vi "Galvo-Control-V2.vi"() -> ()   [LabVIEW 2024]
uses:
  <vilib>/DAQmx/write.llb/DAQmx Write (Analog 1D DBL NChan 1Samp).vi
  <vilib>/DAQmx/create/channels.llb/DAQmx Create Channel (AO-Voltage-Basic).vi
  <vilib>/DAQmx/miscellaneous.llb/DAQmx Fill In Error Info.vi
panel:
  in  "Y desired voltage step(V/100)":dbl=1.0 format="%#_13g"
  in  "X desired voltage step(V/100)":dbl=1.0 format="%#_13g"
  out "Virtual Y position":dbl(graph)
  out "virtual X position":dbl(graph)
  out "Y indic":dbl
  out "X indic.":dbl
  in  "Y origin":dbl
  in  "X origin":dbl
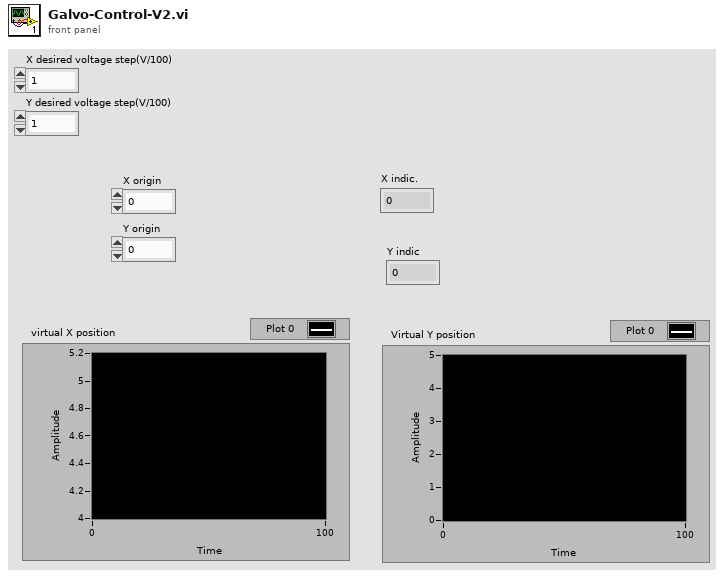
[diagram p1: front panel]
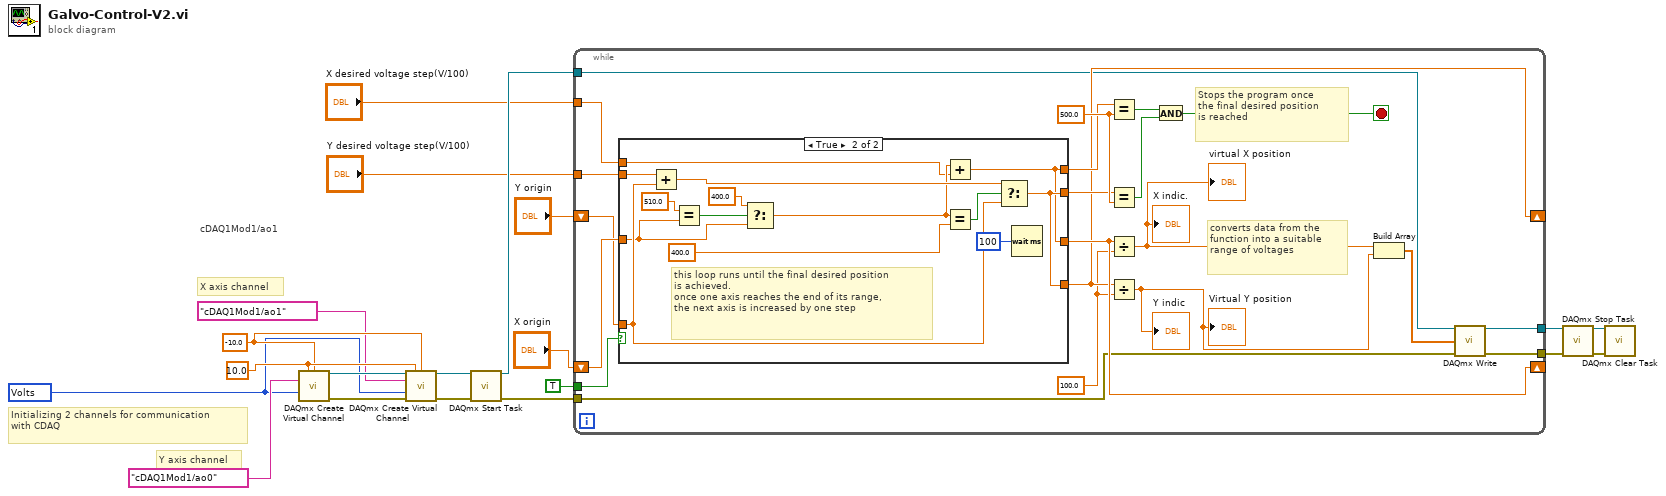
[diagram p0: block diagram]
diagram:
  w8 = 10348 items=["Volts"=10348, "From Custom Scale"=10065] ("units")
  w12 = 10.0 ("maximum value")
  w11 = -10.0 ("minimum value")
  # "Initializing 2 channels for communication\nwith CDAQ"
  # "cDAQ1Mod1/ao1"
  # "X axis channel"
  # "Y axis channel"
  n1 = call-poly <vilib>:"DAQmx Create Virtual Channel.vi"("maximum value"=w12, "minimum value"=w11, "physical channels"=tag "cDAQ1Mod1/ao0", "units"=w8) -> ("task out"=w18:refnum<k21>, "error out"=w17:errorcluster)  [unwired: 10 in]
  n2 = call-poly <vilib>:"DAQmx Create Virtual Channel.vi"("task in"=w18, "maximum value"=w12, "minimum value"=w11, "physical channels"=tag "cDAQ1Mod1/ao1", "units"=w8, "error in"=w17) -> ("task out"=w7:refnum<k21>, "error out"=w6:errorcluster)  [unwired: 8 in]
  n3 = call <vilib>:"DAQmx Start Task.vi"("task/channels in"=w7, "error in"=w6) -> ("task out"=w5:refnum<k21>, "error out"=w4:errorcluster)  [unwired: 12 in]
  n4 = while {
    shift-right: [w32] -> _
    shift-left: "X origin" -> [w41]
    shift-right: [w31] -> _
    shift-left: "Y origin" -> [w40]
    tunnel: TRUE -> [w35]
    tunnel: [w26] -> w16
    tunnel: [w25] -> w15
    tunnel: w5 -> [w24]
    tunnel: w4 -> [w23]
    tunnel: "Y desired voltage step(V/100)" -> [w22]
    tunnel: "X desired voltage step(V/100)" -> [w21]
    stop <- w36 stop-if-true
    w30 = 100.0 ("x")
    w39 = 500.0 ("y")
    # "converts data from the\nfunction into a suitable \nrange of voltages"
    # "Stops the program once\nthe final desired position \nis reached"
    n5 = case shown="True" w35 {
      tunnel: w41 -> [_ w48]
      tunnel: [_ w45] -> w32
      tunnel: w40 -> [_ w49]
      tunnel: [_ w47] -> w31
      tunnel: [_ w45] -> w34
      tunnel: [_ w47] -> w33
      tunnel: w22 -> [_ w43]
      tunnel: w21 -> [_ w42]
      frame False {
      }
      frame True {
        # "this loop runs until the final desired position\nis achieved.\nonce one axis reaches the end of its range,\nthe next axis is increased by one step"
        n6 = Add(x=w43, y=w49) -> (x+y=w50:dbl)
        n7 = Equal?(x=510.0, y=w48) -> (x = y?=w55:bool)
        n8 = Select(t=400.0, s=w55, f=w48) -> (s? t:f=w46:dbl)
        n9 = Add(x=w46, y=w42) -> (x+y=w45:dbl)
        n10 = Equal?(x=w46, y=400.0) -> (x = y?=w51:bool)
        n11 = Select(t=w50, s=w51, f=w49) -> (s? t:f=w47:dbl)
        n12 = Wait (ms)(milliseconds to wait=u32 100) -> ()  [unwired: 1 out]
      }
    }
    n13 = Equal?(x=w34, y=w39) -> (x = y?=w38:bool)
    n14 = Equal?(x=w33, y=w39) -> (x = y?=w37:bool)
    n15 = Divide(x=w32, y=w30) -> (x/y=w28:dbl)
    "X indic." <- w28
    "virtual X position" <- w28
    n16 = Divide(x=w31, y=w30) -> (x/y=w29:dbl)
    "Y indic" <- w29
    "Virtual Y position" <- w29
    n17 = And(x=w38, y=w37) -> (x .and. y?=w36:bool)
    n18 = Build Array(w28, w29) -> (w27:dbl[])
    n19 = call-poly <vilib>:"DAQmx Write.vi"("task/channels in"=w24, "data"=w27, "error in"=w23) -> ("task out"=w26:refnum<k21>, "error out"=w25:errorcluster)  [unwired: 10 in, 1 out]
  }
  n20 = call <vilib>:"DAQmx Stop Task.vi"("task/channels in"=w16, "error in"=w15) -> ("task out"=w14:refnum<k21>, "error out"=w13:errorcluster)  [unwired: 12 in]
  n21 = call <vilib>:"DAQmx Clear Task.vi"("task in"=w14, "error in"=w13) -> ()  [unwired: 13 in, 1 out]
